vi "Check_Sequence.vi"(0 "Input Sequence":cluster{string, string[], dbl[], dbl}[](array[cluster])) -> (1 "Valid Sequence":bool, 2 "Error Indices":i32[](array[numeric]))   [LabVIEW 2011]
doc: "This VI checks a growth sequence for syntax errors. It returns \"True\" if the sequence is valid, otherwise it returns false and displays an error message. If there is an error, it will return the an array of all command indices at which an error occurred."
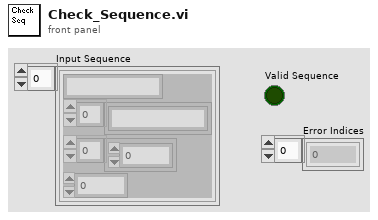
[diagram p1: front panel]
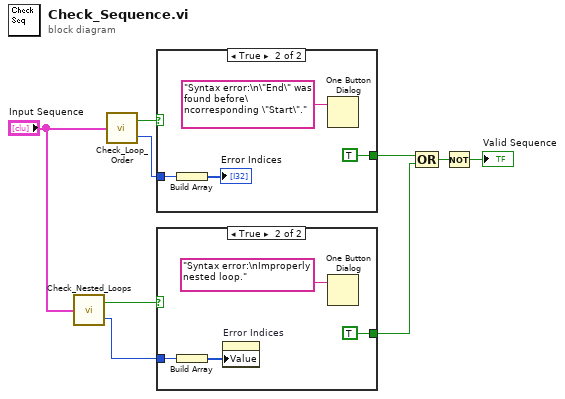
[diagram p0: block diagram]
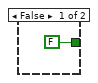
[diagram p2: hidden frame]
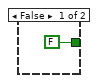
[diagram p3: hidden frame]
diagram:
  n1 = call "Check_Nested_Loops.vi"("Input Sequence"="Input Sequence") -> ("Syntax Error"=w1:bool, "Error Index"=w7:i32)
  n2 = call "Check_Loop_Order.vi"("Input Sequence"="Input Sequence") -> ("Syntax Error"=w9:bool, "Error Index"=w5:i32)
  n3 = case shown="True" w9 {
    tunnel: [FALSE ("true") TRUE ("true")] -> w4
    tunnel: w5 -> [_ w12]
    frame False {
    }
    frame True {
      n4 = Build Array(w12) -> (→"Error Indices":i32[])
      n5 = One Button Dialog(message="Syntax error:\n\"End\" was found before\ncorresponding \"Start\".") -> ()  [unwired: 1 in, 1 out]
    }
  }
  n6 = case shown="True" w1 {
    tunnel: w7 -> [_ w17]
    tunnel: [FALSE ("true") TRUE ("true")] -> w6
    frame False {
    }
    frame True {
      n7 = Build Array(w17) -> (w16:i32[])
      n8 = property on="Error Indices" class="Arr (strict)"("Value"=w16) -> ()  [unwired: 2 in, 2 out]
      n9 = One Button Dialog(message="Syntax error:\nImproperly nested loop.") -> ()  [unwired: 1 in, 1 out]
    }
  }
  n10 = Compound Arithmetic op=OR(w4, w6) -> (w3:bool)
  n11 = Not(x=w3) -> (.not. x?=→"Valid Sequence":bool)
